vi "Actor Core.vi"(8 "error in":errorcluster, 11 "Simulated User Console Actor in":refnum<class "Simulated Sensor Interface Actor.lvclass">) -> (0 "error out":errorcluster, 3 "Actor out":refnum<class "Actor.lvclass">)   [LabVIEW 2019, in "Simulated Sensor Interface Actor.lvlib" / "Simulated Sensor Interface Actor.lvclass"]
doc: "(<B>Filename</B>: Actor Framework.lvlib:Actor.lvclass:Actor Core.vi)\n\nReceives messages to the actor, reacts to them, and initiates any error handling that may shut the actor down.\n\nDescendant classes may override this VI to append parallel tasks for the actor to complete while it handles messages. Overrides use the Call Parent Method node."
uses:
  Simulated Sensor Interface Actor.lvclass
  <vilib>/ActorFramework/Actor/Actor.lvclass
  <vilib>/ActorFramework/Stop Msg/Stop Msg.lvclass
  Sensor Interface Actor/Sensor Interface Actor/Sensor Interface Actor.lvclass
  C:/Workspace/CLA/ATM AF/Sensor Interface Actor/Sensor Interface Actor/Sensor Interface Actor.lvclass
  C:/Program Files (x86)/National Instruments/LabVIEW 2019/vi.lib/ActorFramework/Actor/Actor.lvclass
  ATM Controller/ATM Controller Messages/Deposit Msg/Deposit Msg 2.lvclass
  ATM Controller/ATM Controller Messages/Withdrawal Msg/Withdrawal Msg 2.lvclass
  ATM Controller/ATM Controller Messages/Set Timeout Msg/Set Timeout Msg.lvclass
  ATM Controller/ATM Controller/State -Enum.ctl
  ATM Controller/ATM Controller/ATM Controller.lvclass
panel:
  in  "Funds Dispensed":bool
  in  "Deposit Received":bool
  # "[Covers: UI4] \n[Covers: UI4A] \n[Covers: UI4B]"
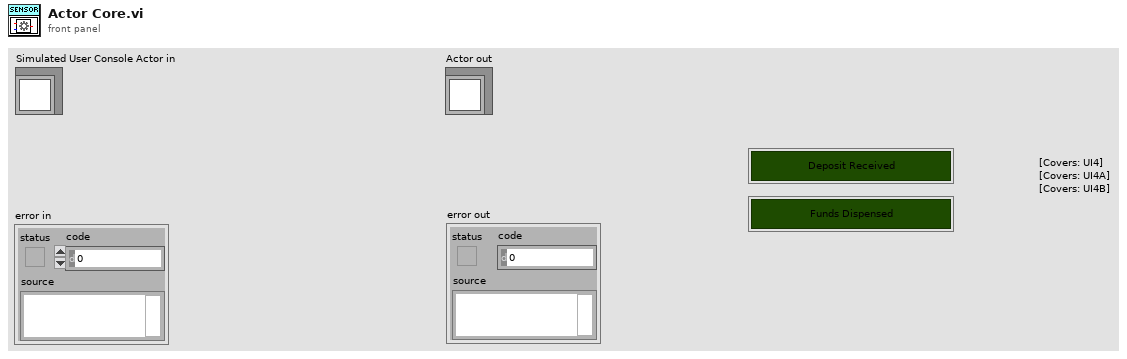
[diagram p1: front panel]
types:
  T1 = typedef "ATM Controller.lvlib/ATM Controller.lvclass/State -Enum.ctl" = enum16{"Inital", "Idle", "Login", "Balance Inquiry", "Deposit", "Withdrawal", "Fast Cash", "Terminate"}
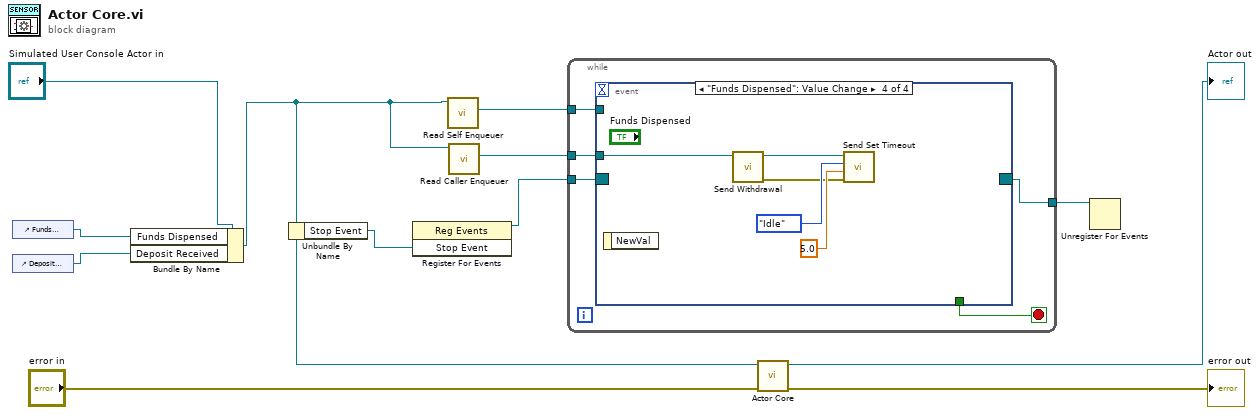
[diagram p0: block diagram]
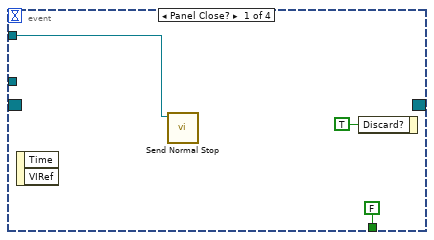
[diagram p2: hidden frame]
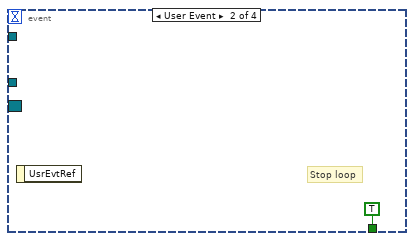
[diagram p3: hidden frame]
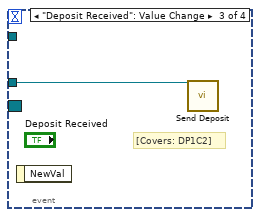
[diagram p4: hidden frame]
diagram:
  n1 = control-ref of="Funds Dispensed"() -> (w4:refnum<vi>)
  n2 = control-ref of="Deposit Received"() -> (w3:refnum<vi>)
  n3 = Bundle By Name(cluster="Simulated User Console Actor in", "Funds Dispensed"=w4, "Deposit Received"=w3) -> (w2:refnum<class "Simulated Sensor Interface Actor.lvclass">)
  n4 = Unbundle By Name(w2) -> ("Stop Event"=w6:refnum<user-event>)
  n5 = register-events(w6) -> (reference out=w8:refnum<event-registration>)  [unwired: 2 in, 1 out]
  n6 = call <vilib>:"Read Self Enqueuer.vi"("Actor"=w2) -> ("Self Enqueuer"=w9:refnum<class "Message Enqueuer.lvclass">)  [unwired: 10 in]
  n7 = call <vilib>:"Read Caller Enqueuer.vi"("Actor"=w2) -> ("Caller Enqueuer"=w1:refnum<class "Message Enqueuer.lvclass">)  [unwired: 10 in]
  n8 = while {
    tunnel: w9 -> [w16]
    tunnel: w8 -> [w15]
    tunnel: [w14] -> w7
    tunnel: w1 -> [w13]
    stop <- w17 stop-if-true
    n9 = event shown="[3] \"Funds Dispensed\": Value Change" {
      selector: w15 -> [_ _ _ _]
      dyn-events: [_ _ _ _] -> w14
      timeout: _ -> [_ _ _ _]
      tunnel: [FALSE TRUE _ _] -> w17
      tunnel: w16 -> [w19 _ _ _]
      tunnel: w13 -> [_ _ w22 w27]
      event Panel Close? {
        n10 = event-data() -> ()  [unwired: 1 in, 2 out]
        n11 = call <vilib>:"Send Normal Stop.vi"("Message Enqueuer"=w19) -> ()  [unwired: 10 in, 1 out]
        n12 = event-data("Discard?"=TRUE) -> ()  [unwired: 1 in, 1 out]
      }
      event User Event {
        # "Stop loop"
        n13 = event-data() -> ()  [unwired: 1 in, 1 out]
      }
      event "Deposit Received": Value Change {
        # "[Covers: DP1C2]"
        n14 = event-data() -> ()  [unwired: 1 in, 1 out]
        n15 = call "Send Deposit.vi"("Message Enqueuer"=w22) -> ()  [unwired: 9 in, 2 out]
      }
      event "Funds Dispensed": Value Change {
        n16 = event-data() -> ()  [unwired: 1 in, 1 out]
        n17 = call "Send Withdrawal.vi"("Message Enqueuer"=w27) -> ("error out"=w23:errorcluster, "Message Enqueuer out"=w26:refnum<class "Message Enqueuer.lvclass">)  [unwired: 9 in]
        n18 = call "Send Set Timeout.vi"("error in (no error)"=w23, "Target Time"=5.0, "State"=State_-Enum."Idle", "Message Enqueuer"=w26) -> ()  [unwired: 6 in, 2 out]
      }
    }
  }
  n19 = call-parent "Actor Core.vi"("error in"="error in", "Actor in"=w2) -> ("error out"=→"error out":errorcluster, "Actor out"=→"Actor out":refnum<class "Actor.lvclass">)  [unwired: 8 in]
  n20 = Unregister For Events(event registration refnum=w7) -> ()  [unwired: 1 in, 1 out]
